vi "Outgoing Page.vi"(8 "error in (no error)":errorcluster, 11 "Node Ptr":T1 format="%.0x") -> (0 "error out":errorcluster)   [LabVIEW 2023, in "Protection and Counter Addon System Explorer.lvlib"]
uses:
  Protection and Counter Addon System Explorer.lvlib
  <vilib>/NI VeriStand/Custom Device API/Custom Device Item Ref.ctl
  SubModules/Frame-Protection-Support/Source/System Explorer/Types/Auto Config Setting.ctl
  Addon Shared/SubVIs/GUID Lookup.vi
  <vilib>/NI VeriStand/Custom Device API/Get Item Property (Variant).vi
  <vilib>/NI VeriStand/Custom Device API/Set Item Property (Variant).vi
  <vilib>/NI VeriStand/Custom Device API/Custom Device API.lvlib
  Addon Shared/Protection and Counter Addon Shared.lvlib
  SubModules/Frame-Protection-Support/Source/System Explorer/Protection and Counter Support System Explorer.lvlib
panel:
  in  "Commit":bool
  in  "CRC Matching Strings":string[](array[string])
  in  "RC Matching Strings":string[](array[string])
  in  "CRC":bool
  in  "Rolling Counter":bool
  in  "SHDocVw.IWebBrowser":refnum<k7>(container)
  in  "Header":cluster{"Section Name":string}={"Section Name"="Auto Config Settings"}
  out "Name":string
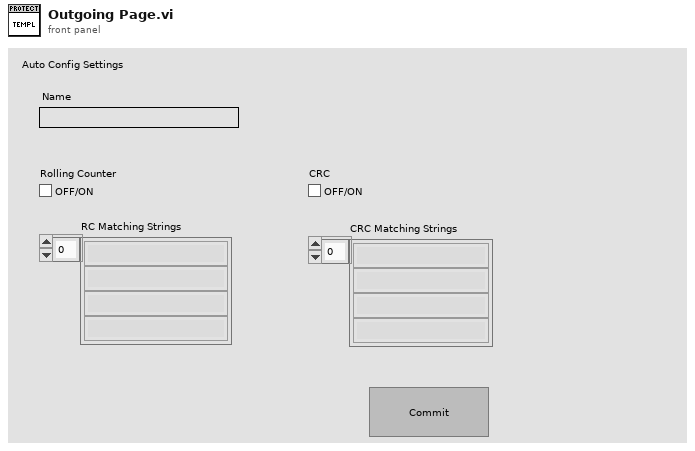
[diagram p1: front panel]
types:
  T1 = typedef "Custom Device API.lvlib/Custom Device Item Ref.ctl" = u64
  T2 = typedef "Protection and Counter Support System Explorer.lvlib/Auto Config Setting.ctl" = cluster{"Rolling Counter":bool, "RC Matching Strings":string[], "CRC":bool, "CRC Matching Strings":string[]}
  T3 = typedef "Custom Device API.lvlib/Custom Device Item Info.ctl" = cluster{"Name":string, "Is Channel":bool, "GUID":string, "Is Waveform":bool}
  T4 = typedef "Custom Device API.lvlib/Custom Device Commands.ctl" = enum16{"Default", "Item renamed", "Shutdown", "Dynamic button pressed"}
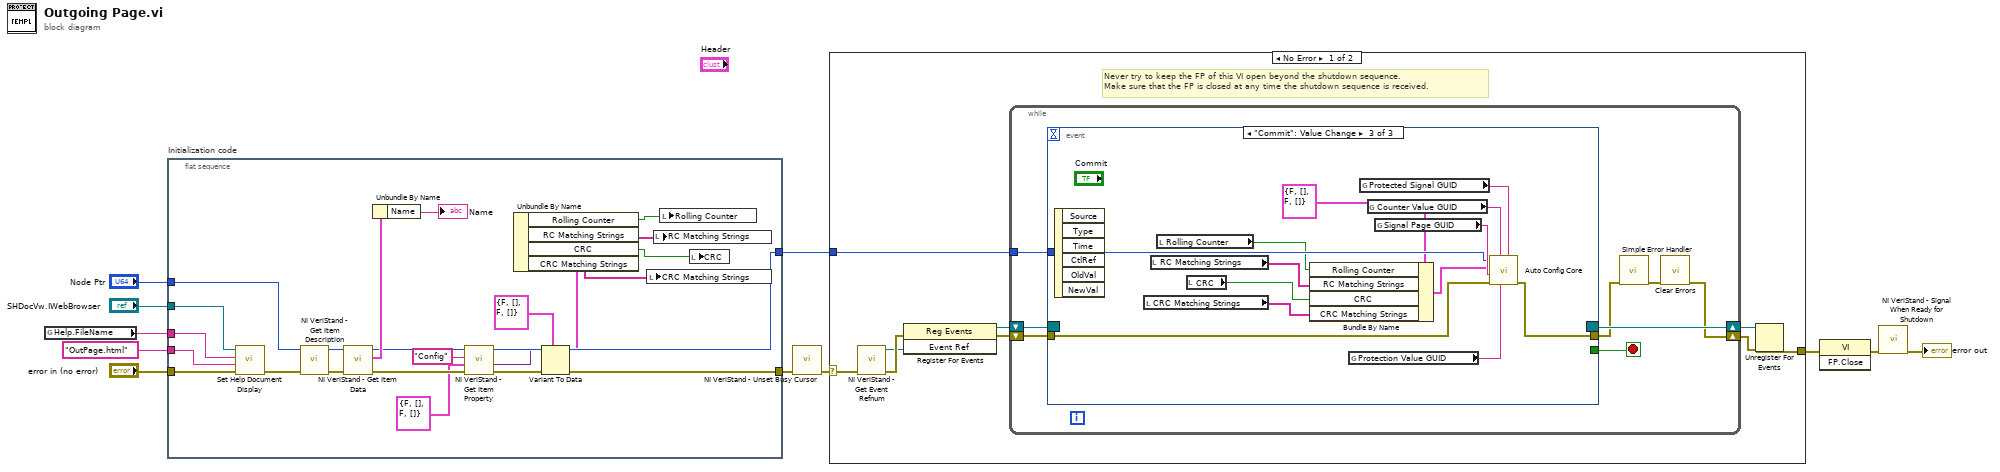
[diagram p0: block diagram]
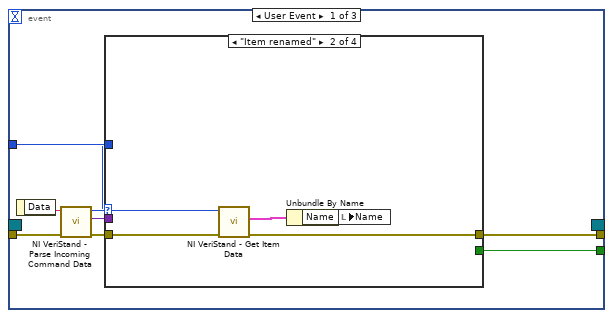
[diagram p2: hidden frame]
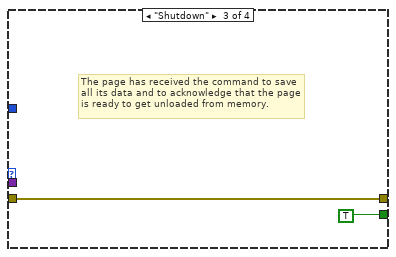
[diagram p4: hidden frame]
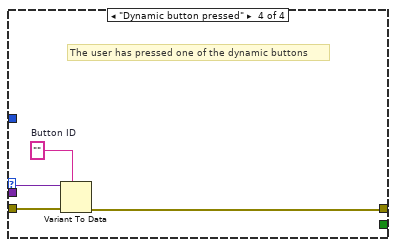
[diagram p5: hidden frame]
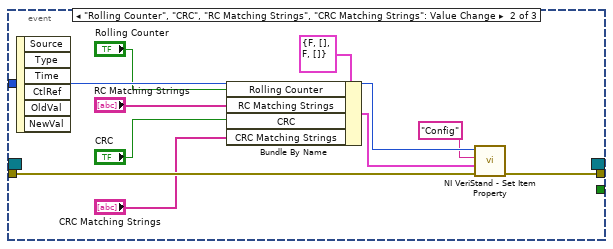
[diagram p6: hidden frame]
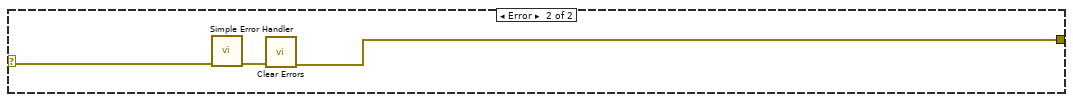
[diagram p7: hidden frame]
diagram:
  n1 = global read "GUID Lookup.vi" "Help.FileName"() -> (w1:string)
  n2 = flat-sequence "Initialization code" {
    tunnel: "error in (no error)" -> [w30]
    tunnel: "Node Ptr" -> [w34]
    tunnel: [w20] -> w7
    tunnel: [w23] -> w4
    tunnel: "OutPage.html" ("HTML File") -> [w28]
    tunnel: w1 -> [w27]
    tunnel: "SHDocVw.IWebBrowser" -> [w26]
    frame #0 {
      n3 = call "Set Help Document Display.vi"("error in (no error)"=w30, "HTML File"=w28, "Main CHM File"=w27, "SHDocVw.IWebBrowser2"=w26) -> ("error out"=w29:errorcluster)  [unwired: 7 in]
      n4 = call <vilib>:"NI VeriStand - Get Item Description.vi"("error in (no error)"=w29, "Item Ref in"=w34) -> ("error out"=w33:errorcluster, "Item Ref out"=w35:T1)  [unwired: 8 out]
      n5 = call <vilib>:"NI VeriStand - Get Item Data.vi"("error in (no error)"=w33, "Item Ref in"=w35) -> ("error out"=w24:errorcluster, "Item Info"=w32:T3, "Item Ref out"=w25:T1)  [unwired: 7 out]
      n6 = Unbundle By Name(w32) -> ("Name"=→"Name":string)
      n7 = call-poly <vilib>:"NI VeriStand - Get Item Property.vi"("error in (no error)"=w24, "Default Value"=T2 {"Rolling Counter"=FALSE, "RC Matching Strings"=[], "CRC"=FALSE, "CRC Matching Strings"=[]} ("Auto Config Setting"), "Property Name"="Config", "Item Ref in"=w25) -> ("error out"=w21:errorcluster, "Value"=w18:variant, "Item Ref out"=w23:T1)  [unwired: 4 in, 1 out]
      n8 = Variant To Data(error in=w21, type=T2 {"Rolling Counter"=FALSE, "RC Matching Strings"=[], "CRC"=FALSE, "CRC Matching Strings"=[]} ("Auto Config Setting"), Variant=w18) -> (data=w17:T2, error out=w20:errorcluster)
      n9 = Unbundle By Name(w17) -> ("Rolling Counter"=w16:bool, "RC Matching Strings"=w15:string[], "CRC"=w14:bool, "CRC Matching Strings"=w13:string[])
      n10 = local write "CRC Matching Strings"(w13) -> ()
      n11 = local write "RC Matching Strings"(w15) -> ()
      n12 = local write "Rolling Counter"(w16) -> ()
      n13 = local write "CRC"(w14) -> ()
    }
  }
  n14 = call <vilib>:"NI VeriStand - Unset Busy Cursor.vi"("error in (no error)"=w7) -> ("error out"=w6:errorcluster)  [unwired: 10 out]
  n15 = case shown="No Error" w6 {
    selector: w6 -> [w36 w98]
    tunnel: [w41 w96] -> w11
    tunnel: w4 -> [w37 _]
    frame No Error {
      # "Never try to keep the FP of this VI open beyond the shutdown sequence.\nMake sure that the FP is closed at any time the shutdown sequence is received."
      n16 = call <vilib>:"NI VeriStand - Get Event Refnum.vi"("error in (no error)"=w36) -> ("error out"=w44:errorcluster, "Event Ref"=w40:refnum<user-event>)  [unwired: 9 out]
      n17 = register-events(error in=w44, w40) -> (reference out=w38:refnum<event-registration>, error out=w39:errorcluster)  [unwired: 1 in]
      n18 = while {
        tunnel: w37 -> [w48]
        shift-right: [w45] -> w42
        shift-left: w39 -> [w51]
        shift-right: [w52] -> w43
        shift-left: w38 -> [w50]
        stop <- w49 stop-if-true
        n19 = event shown="[2] \"Commit\": Value Change" {
          selector: w50 -> [_ _ _]
          dyn-events: [_ _ _] -> w52
          timeout: _ -> [_ _ _]
          tunnel: w51 -> [w60 w81 w91]
          tunnel: [w56 _ _] -> w49
          tunnel: [w55 w80 w92] -> w47
          tunnel: w48 -> [w54 w82 w90]
          event User Event {
            n20 = event-data() -> ("Data"=w59:string)  [unwired: 1 out]
            n21 = call <vilib>:"NI VeriStand - Parse Incoming Command Data.vi"("error in (no error)"=w60, "Incoming data"=w59) -> ("error out"=w58:errorcluster, "Outgoing data"=w53:variant, "Action"=w57:T4)  [unwired: 7 out]
            n22 = case shown="\"Item renamed\"" w57 {
              tunnel: w58 -> [w61 w66 w67 w72]
              tunnel: [_ _ TRUE _] -> w56
              tunnel: [w61 w63 w67 w69] -> w55
              tunnel: w54 -> [_ w65 _ _]
              tunnel: w53 -> [_ _ _ w71]
              frame "Default", Default {
              }
              frame "Item renamed" {
                n23 = call <vilib>:"NI VeriStand - Get Item Data.vi"("error in (no error)"=w66, "Item Ref in"=w65) -> ("error out"=w63:errorcluster, "Item Info"=w64:T3)  [unwired: 8 out]
                n24 = Unbundle By Name(w64) -> ("Name"=w62:string)
                n25 = local write "Name"(w62) -> ()
              }
              frame "Shutdown" {
                # "The page has received the command to save all its data and to acknowledge that the page is ready to get unloaded from memory."
              }
              frame "Dynamic button pressed" {
                w70 = ""  # Button ID
                # "The user has pressed one of the dynamic buttons"
                n26 = Variant To Data(error in=w72, type=w70, Variant=w71) -> (error out=w69:errorcluster)  [unwired: 1 out]
              }
            }
          }
          event "Rolling Counter", "CRC", "RC Matching Strings", "CRC Matching Strings": Value Change {
            n27 = event-data() -> ()  [unwired: 7 out]
            n28 = Bundle By Name(cluster=T2 {"Rolling Counter"=FALSE, "RC Matching Strings"=[], "CRC"=FALSE, "CRC Matching Strings"=[]} ("Auto Config Setting"), "Rolling Counter"="Rolling Counter", "RC Matching Strings"="RC Matching Strings", "CRC"="CRC", "CRC Matching Strings"="CRC Matching Strings") -> (w73:T2)
            n29 = call-poly <vilib>:"NI VeriStand - Set Item Property.vi"("error in (no error)"=w81, "Value"=w73, "Property Name"="Config", "Item Ref in"=w82) -> ("error out"=w80:errorcluster)  [unwired: 5 in, 2 out]
          }
          event "Commit": Value Change {
            n30 = event-data() -> ()  [unwired: 7 out]
            n31 = local read "CRC Matching Strings"() -> (w85:string[])
            n32 = local read "RC Matching Strings"() -> (w87:string[])
            n33 = local read "Rolling Counter"() -> (w89:bool)
            n34 = local read "CRC"() -> (w86:bool)
            n35 = Bundle By Name(cluster=T2 {"Rolling Counter"=FALSE, "RC Matching Strings"=[], "CRC"=FALSE, "CRC Matching Strings"=[]} ("Auto Config Setting"), "Rolling Counter"=w89, "RC Matching Strings"=w87, "CRC"=w86, "CRC Matching Strings"=w85) -> (w84:T2)
            n36 = global read "GUID Lookup.vi" "Protection Value GUID"() -> (w83:string)
            n37 = global read "GUID Lookup.vi" "Protected Signal GUID"() -> (w93:string)
            n38 = global read "GUID Lookup.vi" "Counter Value GUID"() -> (w94:string)
            n39 = global read "GUID Lookup.vi" "Signal Page GUID"() -> (w95:string)
            n40 = call "Auto Config Core.vi"("Protected Signal GUID"=w93, "Protection Value GUID"=w83, "Counter Value GUID"=w94, "error in (no error)"=w91, "Signal Page GUID"=w95, "Auto Config Setting"=w84, "Node Ptr"=w90) -> ("error out"=w92:errorcluster)  [unwired: 4 in]
          }
        }
        n41 = call <vilib>:"Simple Error Handler.vi"("error in (no error)"=w47) -> ("error out"=w46:errorcluster)  [unwired: 1 in, 7 out]
        n42 = call <vilib>:"Clear Errors.vi"("error in (no error)"=w46) -> ("error out"=w45:errorcluster)  [unwired: 1 in, 5 out]
      }
      n43 = Unregister For Events(event registration refnum=w43, error in=w42) -> (error out=w41:errorcluster)
    }
    frame Error {
      n44 = call <vilib>:"Simple Error Handler.vi"("error in (no error)"=w98) -> ("error out"=w97:errorcluster)  [unwired: 1 in, 7 out]
      n45 = call <vilib>:"Clear Errors.vi"("error in (no error)"=w97) -> ("error out"=w96:errorcluster)  [unwired: 1 in, 5 out]
    }
  }
  n46 = invoke class="VI" method="FP.Close"(error in=w11) -> (error out=w10:errorcluster)  [unwired: 2 in, 2 out]
  n47 = call <vilib>:"NI VeriStand - Signal When Ready for Shutdown.vi"("error in (no error)"=w10) -> ("error out"=→"error out":errorcluster)  [unwired: 10 out]
